vi "n_edge.vi"(11 "In":bool) -> (3 "Out":bool)   [LabVIEW 2013]
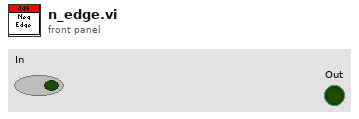
[diagram p1: front panel]
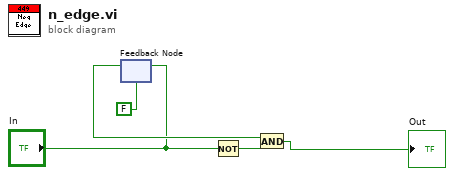
[diagram p0: block diagram]
diagram:
  n1 = feedback-in #1("In") -> ()
  n2 = feedback #1(FALSE ("In")) -> (w5:bool)
  n3 = Not(x="In") -> (.not. x?=w4:bool)
  n4 = And(x=w5, y=w4) -> (x .and. y?=→"Out":bool)
